vi "Virtual_Sensors.vi"() -> ()   [LabVIEW 2026]
panel:
  out "Status":string
  out "Sequence Number":dbl
  out "Last Packet Sent":string
  in  "SEND ALL":bool
  in  "Downstream Rise":dbl
  in  "Upstream Rise":dbl
  in  "Tilt Change":dbl
  in  "Soil Moisture":dbl
  in  "Rainfall":dbl
  in  "ZONE ID":string
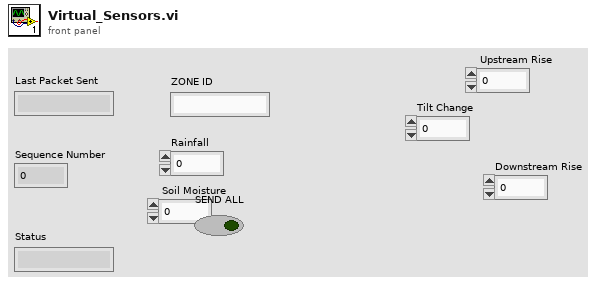
[diagram p1: front panel]
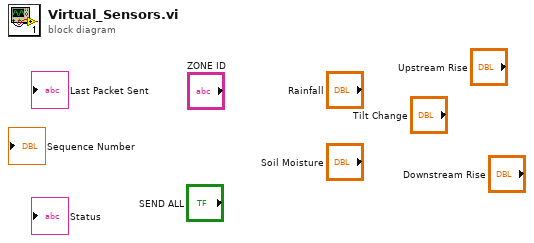
[diagram p0: block diagram]
diagram:
